vi "error deadtime.vi"(1 "deadtime":dbl) -> (0 "dead time error":dbl)   [LabVIEW 2016]
doc: "This calculates the dead time portion of the internal error"
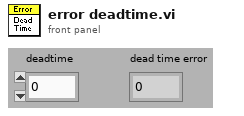
[diagram p1: front panel]
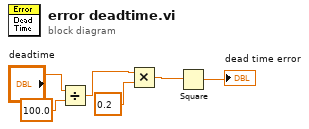
[diagram p0: block diagram]
diagram:
  n1 = Divide(x="deadtime", y=100.0) -> (x/y=w2:dbl)
  n2 = Multiply(x=w2, y=0.2) -> (x*y=w5:dbl)
  n3 = Square(x=w5) -> (x^2=→"dead time error":dbl)
